vi "initAque.vi"(8 "error in (no error)":errorcluster, 11 "IVI Refnum in":refnum<k15>) -> (0 "error out":errorcluster, 3 "IVI Refnum out":refnum<k15>)   [LabVIEW 2011]
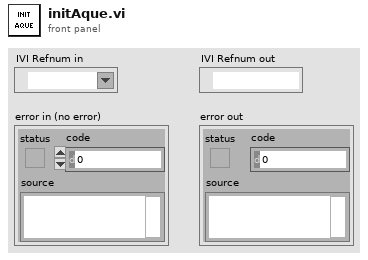
[diagram p1: front panel]
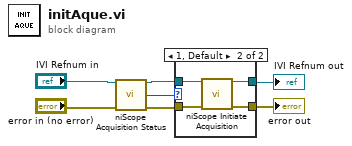
[diagram p0: block diagram]
diagram:
  n1 = call "niScope Acquisition Status.vi"("instrument handle"="IVI Refnum in", "error in"="error in (no error)") -> ("instrument handle out"=w4:refnum<k15>, "acquisition status"=w5:i32, "error out"=w7:errorcluster)  [unwired: 11 in]
  n2 = case shown="1, Default" w5 {
    tunnel: [w9 w13] -> w1
    tunnel: [w8 w12] -> w2
    tunnel: w7 -> [w8 w11]
    tunnel: w4 -> [w9 w10]
    frame 0 {
    }
    frame 1, Default {
      n3 = call "niScope Initiate Acquisition.vi"("instrument handle"=w10, "error in"=w11) -> ("instrument handle out"=w13:refnum<k15>, "error out"=w12:errorcluster)  [unwired: 12 in]
    }
  }
  "error out" <- w2
  "IVI Refnum out" <- w1
